vi "Act2_recibir.vi"() -> ()   [LabVIEW 2020]
uses:
  <vilib>/httpClient/LabVIEWHTTPClient.lvlib
panel:
  out "headers 2":string
  out "body 2":string
  out "error out 2":errorcluster
  out "Tempreratura":dbl
  out "Frontal":bool
  out "Lateral":bool
  out "error out":errorcluster
  in  "stop":bool
  out "Fecha":string
  out "Humedad":dbl
  out "body":string
  out "headers":string
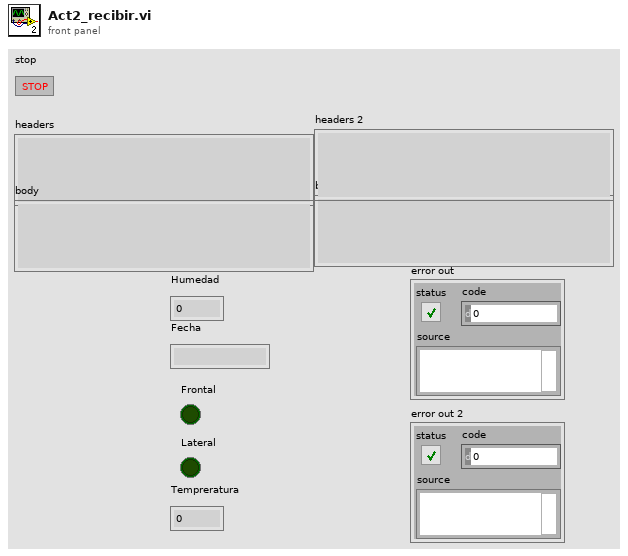
[diagram p1: front panel]
types:
  T1 = cluster{"Frontal":bool, "Lateral":bool, "Temperatura":dbl}
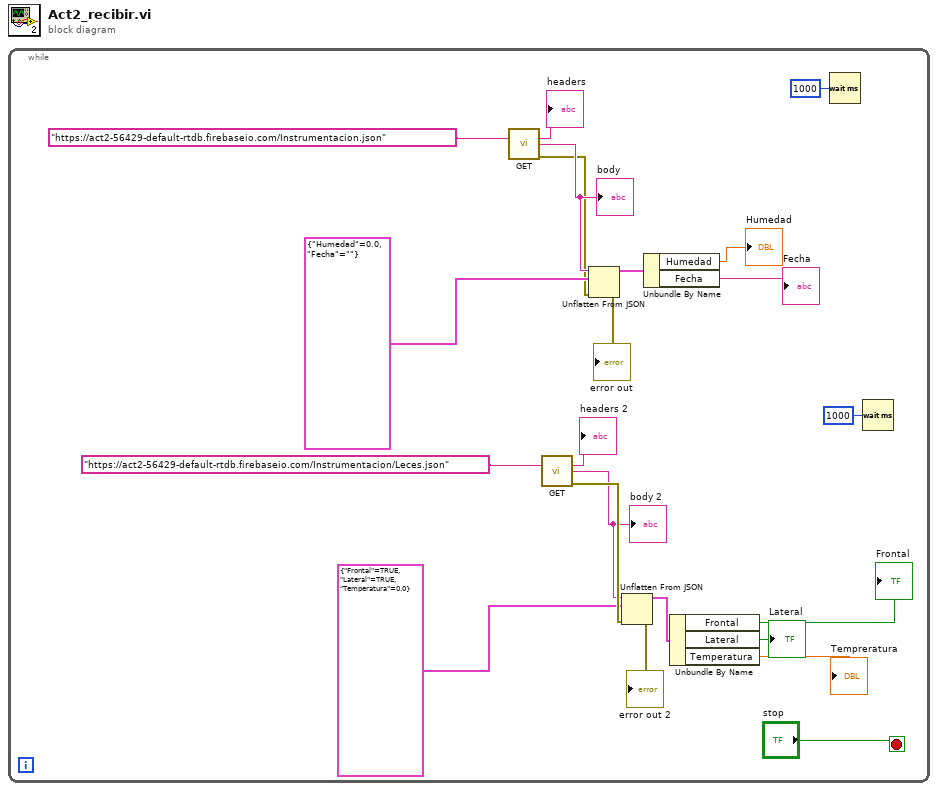
[diagram p0: block diagram]
diagram:
  n1 = while {
    stop <- "stop" stop-if-true
    n2 = call <vilib>:"GET.vi"("url"="https://act2-56429-default-rtdb.firebaseio.com/Instrumentacion.json" ("string")) -> ("headers"=→"headers":string, "body"=w20:string, "error out"=w14:errorcluster)  [unwired: 11 in, 1 out]
    "body" <- w20
    n3 = call <vilib>:"GET.vi"("url"="https://act2-56429-default-rtdb.firebaseio.com/Instrumentacion/Leces.json" ("string")) -> ("headers"=→"headers 2":string, "body"=w3:string, "error out"=w6:errorcluster)  [unwired: 11 in, 1 out]
    "body 2" <- w3
    n4 = Unflatten From JSON(JSON string=w20, type and defaults=cluster{"Humedad":dbl, "Fecha":string} {"Humedad"=0.0, "Fecha"=""}, error in (no error)=w14) -> (value=w19:cluster{"Humedad":dbl, "Fecha":string}, error out=→"error out":errorcluster)  [unwired: 4 in]
    n5 = Unflatten From JSON(JSON string=w3, type and defaults=T1 {"Frontal"=TRUE, "Lateral"=TRUE, "Temperatura"=0.0}, error in (no error)=w6) -> (value=w4:T1, error out=→"error out 2":errorcluster)  [unwired: 4 in]
    n6 = Unbundle By Name(w19) -> ("Humedad"=→"Humedad":dbl, "Fecha"=→"Fecha":string)
    n7 = Unbundle By Name(w4) -> ("Frontal"=→"Frontal":bool, "Lateral"=→"Lateral":bool, "Temperatura"=→"Tempreratura":dbl)
    n8 = Wait (ms)(milliseconds to wait=u32 1000) -> ()  [unwired: 1 out]
    n9 = Wait (ms)(milliseconds to wait=u32 1000) -> ()  [unwired: 1 out]
  }
